vi "Read Timestamp.vi"(8 "error in (no error)":errorcluster, 11 "MsgPackTimestamp in":refnum<class "MsgPackTimestamp.lvclass">) -> (0 "error out":errorcluster, 2 "Timestamp":timestamp, 3 "MsgPackTimestamp out":refnum<class "MsgPackTimestamp.lvclass">)   [LabVIEW 2020, in "MessagePack.lvlib" / "MsgPackTimestamp.lvclass"]
uses:
  MsgPackTimestamp.lvclass
  MsgPackTimestamp.lvclass/MsgPackTimestamp.ctl
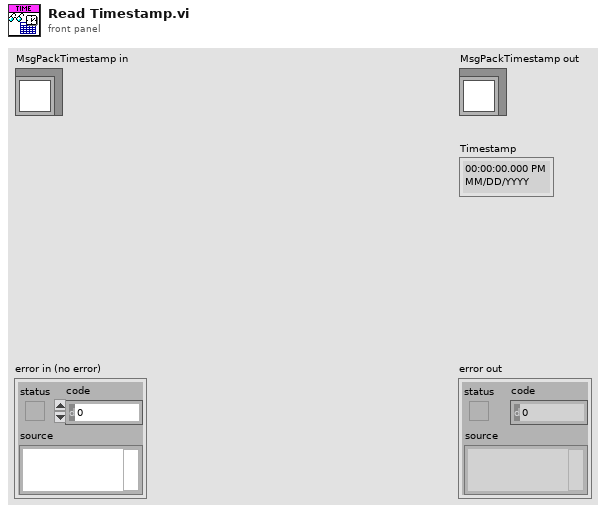
[diagram p1: front panel]
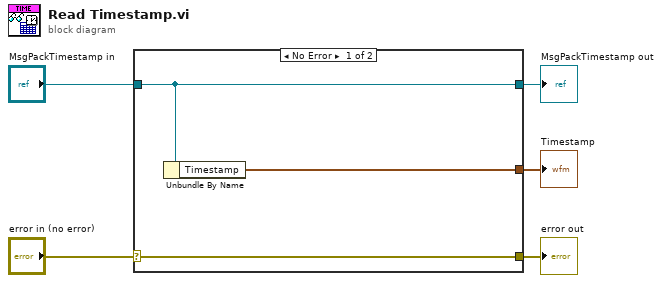
[diagram p0: block diagram]
diagram:
  n1 = case shown="No Error" "error in (no error)" {
    selector: "error in (no error)" -> [w8 w9]
    tunnel: [w8 w9] -> w4
    tunnel: [w7 w10] -> w2
    tunnel: "MsgPackTimestamp in" -> [w7 w10]
    tunnel: [w6 _] -> w1
    frame No Error {
      n2 = Unbundle By Name(w7) -> ("Timestamp"=w6:timestamp)
    }
    frame Error {
    }
  }
  "error out" <- w4
  "MsgPackTimestamp out" <- w2
  "Timestamp" <- w1
